vi "XWPF Writer - Append Text Tests.vi"() -> (3 "All Paragraphs":string[](array[string]), 5 "Text":string)   [LabVIEW 2017]
uses:
  src/Styles/Alignment--ring.ctl
  src/Styles/Underline--ring.ctl
  src/Styles/Style/Get Style Name.vi
  src/Styles/Style/Style.lvclass
  src/LabVIEW NPOI/xwpfWriter/xwpfWriter.lvclass
  src/Styles/Heading 3/Heading 3.lvclass
  src/LabVIEW NPOI/xwpfReader/xwpfReader.lvclass
  C:/Users/Neo/Desktop/Dev_Tools_BR/LabVIEW_NPOI/src/Styles/Style/Style.lvclass
  src/Styles/Styles.lvlib
panel:
  out "Array 6":string[](array[string])
  out "Array 5":T1[](array[typedef]) items=["Single"=1, "Words"=2, "Double"=3, "Thick"=4, "Dotted"=5, "DottedHeavy"=6, "Dash"=7, "DashedHeavy"=8, "DashLong"=9, "DashLongHeavy"=10, "DotDash"=11, "DashDotHeavy"=12, "DotDotDash"=13, "DashDotDotHeavy"=14, "Wave"=15, "WavyHeavy"=16, "WavyDouble"=17, "None"=18]
  out "Array 4":T2[](array[typedef]) items=["LEFT"=1, "CENTER"=2, "RIGHT"=3, "BOTH"=4, "MEDIUM_KASHIDA"=5, "DISTRIBUTE"=6, "NUM_TAB"=7, "HIGH_KASHIDA"=8, "LOW_KASHIDA"=9, "THAI_DISTRIBUTE"=10]
  out "Array 3":u32[](array[colorbox])
  out "Array 2":i32[](array[numeric])
  out "Array":string[](array[string])
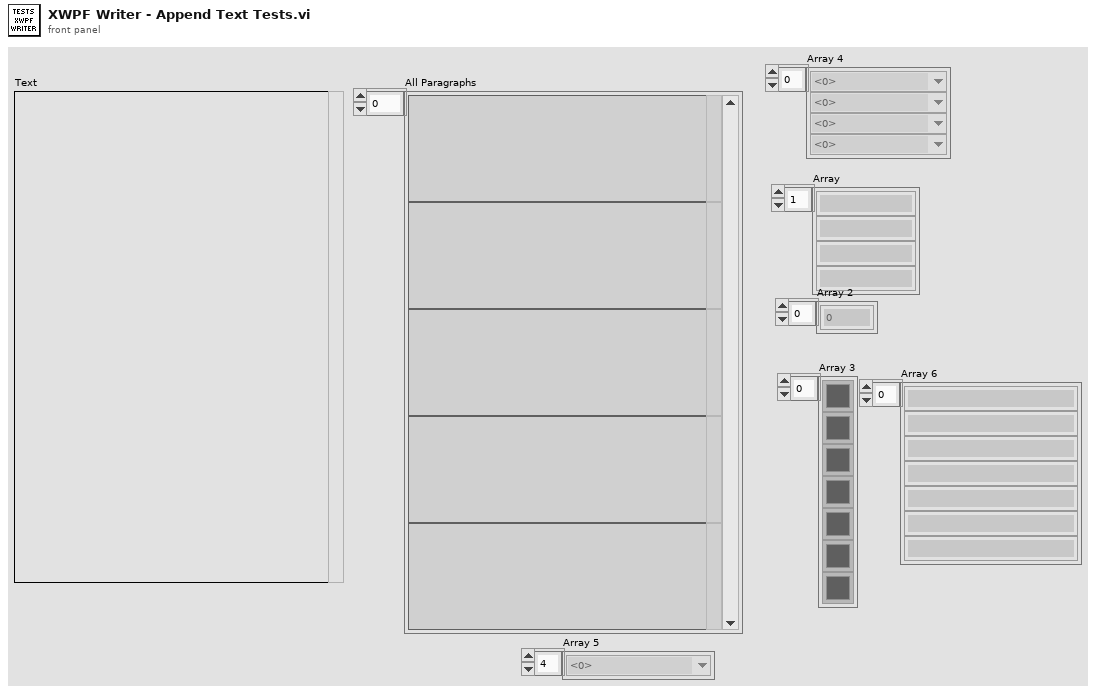
[diagram p1: front panel]
types:
  T1 = typedef "Styles.lvlib/Underline--ring.ctl" = i32
  T2 = typedef "Styles.lvlib/Alignment--ring.ctl" = i32
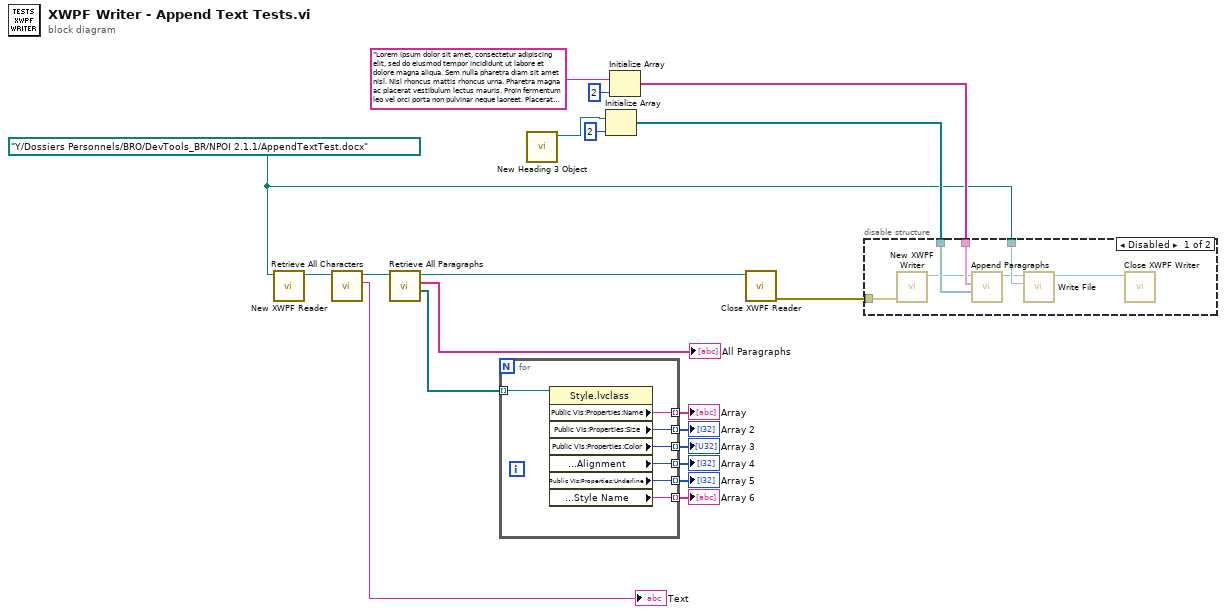
[diagram p0: block diagram]
diagram:
  w8 = path "Y:/Dossiers Personnels/BRO/DevTools_BR/NPOI 2.1.1/AppendTextTest.docx" ("path")
  n1 = call "New XWPF Reader.vi"("XWPF File Path"=w8) -> ("xwpfReader out"=w14:refnum<class "xwpfReader.lvclass">)  [unwired: 9 in, 1 out]
  n2 = call "Retrieve All Characters.vi"("xwpfReader in"=w14) -> ("All Characters"=→"Text":string, "xwpfReader out"=w13:refnum<class "xwpfReader.lvclass">)  [unwired: 8 in, 1 out]
  n3 = call "Retrieve All Paragraphs.vi"("xwpfReader in"=w13) -> ("Paragraph Styles"=w7:refnum<class "Style.lvclass">[], "Paragraphs"=→"All Paragraphs":string[], "xwpfReader out"=w12:refnum<class "xwpfReader.lvclass">)  [unwired: 7 in, 1 out]
  n4 = for {
    tunnel: w7 -> [w27] mode=indexing
    tunnel: [w26] -> w6 mode=indexing
    tunnel: [w25] -> w5 mode=indexing
    tunnel: [w24] -> w4 mode=indexing
    tunnel: [w23] -> w3 mode=indexing
    tunnel: [w22] -> w2 mode=indexing
    tunnel: [w21] -> w1 mode=indexing
    n5 = property class="Style.lvclass"(reference=w27) -> ("Public VIs:Properties:Name"=w26:string, "Public VIs:Properties:Size"=w25:i32, "Public VIs:Properties:Color"=w24:u32, "Public VIs:Properties:Alignment"=w23:T2, "Public VIs:Properties:Underline"=w22:T1, "Public VIs:Properties:Style Name"=w21:string)  [unwired: 1 in, 2 out]
  }
  "Array" <- w6
  "Array 2" <- w5
  "Array 3" <- w4
  "Array 4" <- w3
  "Array 5" <- w2
  "Array 6" <- w1
  n6 = call "New Heading 3 Object.vi"() -> ("Heading 3 out"=w18:refnum<class "Heading 3.lvclass">)  [unwired: 10 in, 1 out]
  n7 = Initialize Array(w18, 2 ("dimension size")) -> (w16:refnum<class "Heading 3.lvclass">[])
  n8 = Initialize Array("Lorem ipsum dolor sit amet, consectetur adipiscing elit, sed do eiusmod tempor incididunt ut labore et dolore magna aliqua. Sem nulla pharetra diam sit amet nisl. Nisl rhoncus mattis rhoncus urna. Pharetra magna ac placerat vestibulum lectus mauris. Proin fermentum leo vel orci porta non pulvinar neque laoreet. Placerat duis ultricies lacus sed turpis tincidunt id aliquet risus. Turpis egestas sed tempus urna et pharetra pharetra. Tellus mauris a diam maecenas sed enim ut sem viverra. Eget mi proin sed libero enim sed. Nunc eget lorem dolor sed viverra ipsum nunc aliquet. Diam vulputate ut pharetra sit amet aliquam id diam. Turpis massa tincidunt dui ut ornare lectus. Ultrices eros in cursus turpis massa tincidunt. Tristique risus nec feugiat in fermentum posuere urna nec tincidunt." ("Text"), 2 ("dimension size")) -> (w15:string[])
  n9 = call "Close XWPF Reader.vi"("xwpfReader in"=w12) -> ("error out"=w11:errorcluster)  [unwired: 9 in, 1 out]
  n10 = disable-structure shown="Disabled" {
    disable-tunnel: w16 -> [w33 _]
    disable-tunnel: w15 -> [w32 _]
    disable-tunnel: w11 -> [w30 _]
    disable-tunnel: w8 -> [w29 _]
    frame Disabled {
      n11 = call "New XWPF Writer.vi"("error in (no error)"=w30) -> ("xwpfWriter out"=w31:refnum<class "xwpfWriter.lvclass">)  [unwired: 9 in, 1 out]
      n12 = call "Append Paragraphs.vi"("Styles"=w33, "Paragraphs"=w32, "xwpfWriter in"=w31) -> ("xwpfWriter out"=w28:refnum<class "xwpfWriter.lvclass">)  [unwired: 7 in, 1 out]
      n13 = call "Write File.vi"("path"=w29, "xwpfWriter in"=w28) -> ("xwpfWriter out"=w34:refnum<class "xwpfWriter.lvclass">)  [unwired: 8 in, 1 out]
      n14 = call "Close XWPF Writer.vi"("xwpfWriter in"=w34) -> ()  [unwired: 9 in, 2 out]
    }
    frame Enabled {
    }
  }
